vi "Read track.vi"() -> ()   [LabVIEW 2017]
panel:
  out "value":T1(array[cluster])
  out "text":string
  in  "file (use dialog)":path=path "D:/upwork/urartu project/urartu/tracks/track_0_minsk.json"
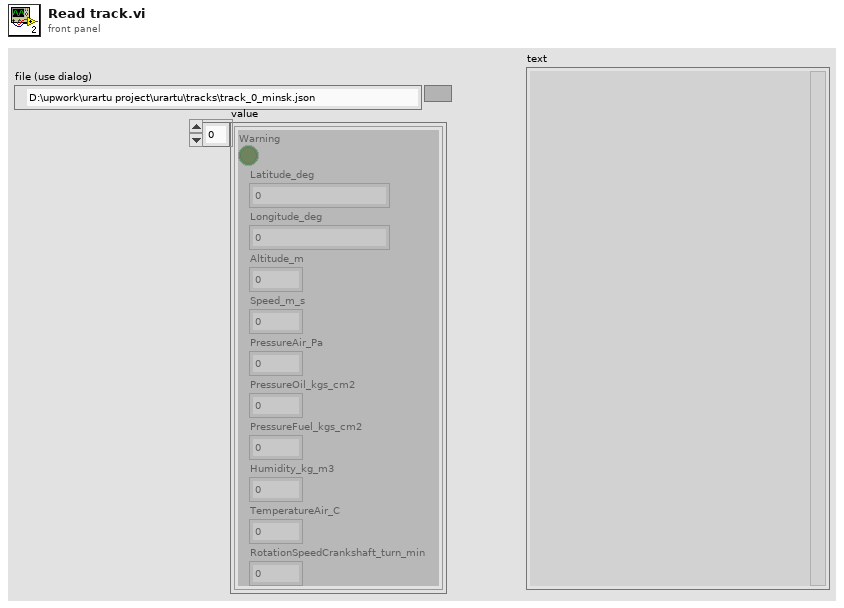
[diagram p1: front panel]
types:
  T1 = cluster{"Warning":bool, "Latitude_deg":dbl, "Longitude_deg":dbl, "Altitude_m":dbl, "Speed_m_s":dbl, "PressureAir_Pa":dbl, "PressureOil_kgs_cm2":dbl, "PressureFuel_kgs_cm2":dbl, "Humidity_kg_m3":dbl, "TemperatureAir_C":dbl, "RotationSpeedCrankshaft_turn_min":dbl}[]
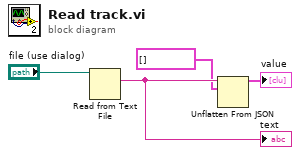
[diagram p0: block diagram]
diagram:
  n1 = Read from Text File(file (use dialog)="file (use dialog)") -> (text=w3:string)  [unwired: 3 in, 3 out]
  "text" <- w3
  n2 = Unflatten From JSON(JSON string=w3, type and defaults=T1 []) -> (value=→"value":T1)  [unwired: 5 in, 1 out]
